vi "ID To Timing and Sync Device.vi"(8 "error in (no error)":errorcluster, 11 "ID in":T1 format="%.0x") -> (0 "error out":errorcluster, 2 "Device":refnum<k24>, 3 "ID out":u64 format="%.0x")   [LabVIEW 2020, in "Custom Device Offline API.lvlib"]
uses:
  <vilib>/NI VeriStand/Custom Device Offline API/Custom Device Offline API.lvlib
  <vilib>/NI VeriStand/Custom Device API/Custom Device Item Ref.ctl
  NationalInstruments.VeriStand.SystemDefinitionAPI
  <vilib>/NI VeriStand/Custom Device API/Custom Device API.lvlib
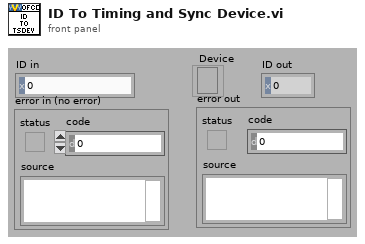
[diagram p1: front panel]
types:
  T1 = typedef "Custom Device API.lvlib/Custom Device Item Ref.ctl" = u64
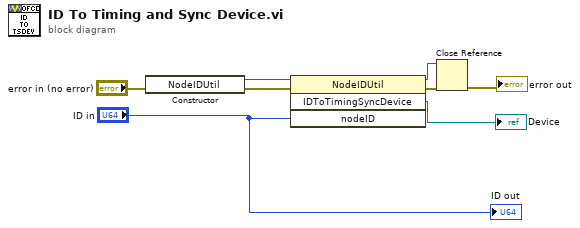
[diagram p0: block diagram]
diagram:
  n1 = constructor class="NodeIDUtil"(error in="error in (no error)") -> (reference out=w8:refnum<k24>, error out=w7:errorcluster)  [unwired: 2 in, 1 out]
  n2 = invoke class="NodeIDUtil" method="IDToTimingSyncDevice"(reference=w8, error in=w7, "nodeID"="ID in") -> (reference out=w4:refnum<k24>, error out=w5:errorcluster, "IDToTimingSyncDevice"=→"Device":refnum<k24>)  [unwired: 1 in, 1 out]
  n3 = Close Reference(reference=w4, error in (no error)=w5) -> (error out=→"error out":errorcluster)
  "ID out" <- "ID in"
